vi "FTW-CodeGen-UpdateStateWithRef.vi"(0 "Old State":variant, 5 "XRef":refnum<vi>, 7 "Version":T1) -> (4 "State Out":T2 {"Width" format="%dpx"}, 6 "Reply":string[](array[string]), 8 "Is Good?":bool)   [LabVIEW 2015, in "FTW-Dataflow-Burrow.xnode"]
uses:
  FTW-Dataflow-Burrow.xnode
  FTW-CodeGen-State.ctl
panel:
  # "Inputs"
  # "Outputs"
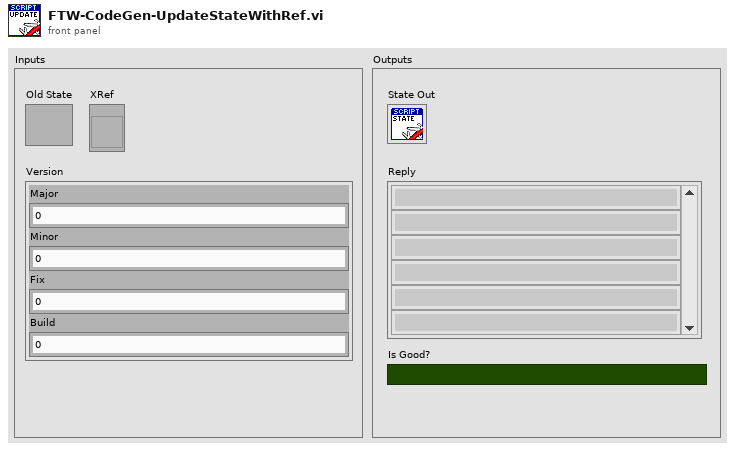
[diagram p1: front panel]
types:
  T1 = cluster{"Major":u16, "Minor":u16, "Fix":u16, "Build":u16}
  T2 = typedef "FTW-Dataflow-Burrow.xnode/FTW-CodeGen-State.ctl" = cluster{"InputTerminals":cluster{"Wired?":bool, "ID":string, "DataName":string, "DataColor":u32, "Type":variant}[], "EnableTiming?":bool, "Width":i32}
  T3 = cluster{"InputTerminals":cluster{"Wired?":bool, "ID":string, "DataName":string, "DataColor":u32, "Type":variant}[], "EnableTiming?":bool}
  T4 = cluster{"Wired?":bool, "ID":string, "DataName":string, "DataColor":u32, "Type":variant}[]
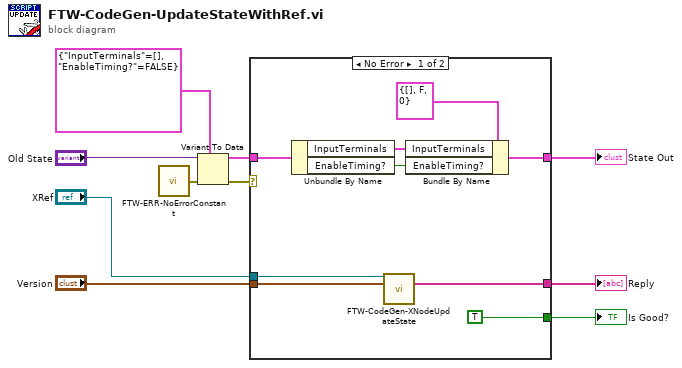
[diagram p0: block diagram]
diagram:
  n1 = call "FTW-ERR-NoErrorConstant.vi"() -> ("no error"=w5:errorcluster)
  n2 = Variant To Data(error in=w5, type=T3 {"InputTerminals"=[], "EnableTiming?"=FALSE} ("State Out"), Variant="Old State") -> (data=w3:T3, error out=w2:errorcluster)
  n3 = case shown="No Error" w2 {
    tunnel: [TRUE ("Is Good?") _] -> w10
    tunnel: "Version" -> [w18 _]
    tunnel: "XRef" -> [w17 _]
    tunnel: [w16 _] -> w7
    tunnel: w3 -> [w15 _]
    tunnel: [w13 _] -> w1
    frame No Error {
      n4 = Unbundle By Name(w15) -> ("InputTerminals"=w12:T4, "EnableTiming?"=w11:bool)
      n5 = call "FTW-CodeGen-XNodeUpdateState.vi"("XRef"=w17, "Previous Version"=w18) -> ("Reply"=w16:string[])  [unwired: 13 in]
      n6 = Bundle By Name(cluster=T2 {"InputTerminals"=[], "EnableTiming?"=FALSE, "Width"=0} ("State Out"), "InputTerminals"=w12, "EnableTiming?"=w11) -> (w13:T2)
    }
    frame Error {
    }
  }
  "State Out" <- w1
  "Reply" <- w7
  "Is Good?" <- w10
